vi "Network Streams Chat Window Launcher.vi"() -> ()   [LabVIEW 2020]
uses:
  Chat Window/Chat Window.lvclass
  <vilib>/ActorFramework/Actor/Actor.lvclass
  <vilib>/ni/Actors/Network Endpoint Actors/Protocols/Network Stream Strategy/Netowrk Stream Listener/Network Stream Listener.lvclass
  <vilib>/ni/Actors/Network Endpoint Actors/Protocols/Network Stream Strategy/Network Stream Initiator/Network Stream Initiator.lvclass
panel:
  in  "Listener Name":string="Bob"
  in  "Address":string="127.0.0.1"
  in  "Initiator Name":string="Fred"
  out "error out":errorcluster
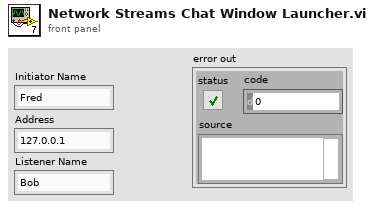
[diagram p1: front panel]
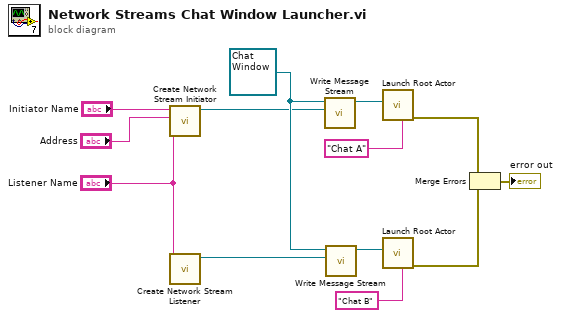
[diagram p0: block diagram]
diagram:
  w13 = refnum<class "Chat Window.lvclass"> refnum ("Chat Window in")
  n1 = call <vilib>:"Create Network Stream Initiator.vi"("Remote Name"="Listener Name", "Remote Address"="Address", "Name"="Initiator Name") -> ("Network Stream Initiator out"=w5:refnum<class "Network Stream Initiator.lvclass">)  [unwired: 8 in]
  n2 = call <vilib>:"Create Network Stream Listener.vi"("Name"="Listener Name") -> ("Network Stream Listener"=w4:refnum<class "Network Stream Listener.lvclass">)  [unwired: 10 in]
  n3 = call "Write Message Stream.vi"("Message Stream"=w5, "Chat Window in"=w13) -> ("Chat Window out"=w12:refnum<class "Chat Window.lvclass">)  [unwired: 9 in]
  n4 = call "Write Message Stream.vi"("Message Stream"=w4, "Chat Window in"=w13) -> ("Chat Window out"=w6:refnum<class "Chat Window.lvclass">)  [unwired: 9 in]
  n5 = call <vilib>:"Launch Root Actor.vi"("Debug Alias"="Chat A", "Actor"=w12) -> ("error out"=w9:errorcluster)  [unwired: 8 in, 1 out]
  n6 = call <vilib>:"Launch Root Actor.vi"("Debug Alias"="Chat B", "Actor"=w6) -> ("error out"=w8:errorcluster)  [unwired: 8 in, 1 out]
  n7 = Merge Errors(w9, w8) -> (→"error out":errorcluster)
